vi "ArrayToExcelColumns.vi"(8 "error in (no error)":errorcluster, 9 "start row":i32, 10 "ArrayData":string[](array[string]), 11 "report in":refnum<class "NI_report.lvclass">) -> (0 "error in (no error) 2":errorcluster, 3 "report in 2":refnum<class "NI_report.lvclass">)   [LabVIEW 2012]
uses:
  <vilib>/Utility/NIReport.llb/NI_report.lvclass
  <vilib>/Utility/NIReport.llb/Excel/NI_Excel.lvclass
panel:
  in  "?":cluster{"start row":i32, "start column":i32}
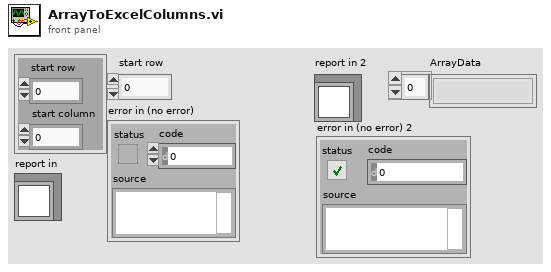
[diagram p1: front panel]
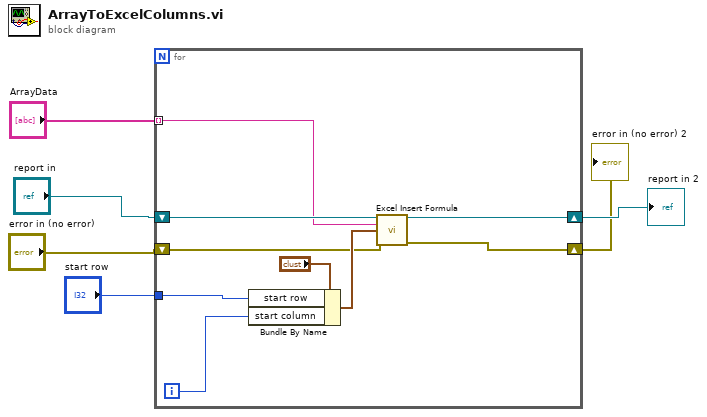
[diagram p0: block diagram]
diagram:
  n1 = for {
    tunnel: "start row" -> [w13]
    shift-right: [w11] -> w2
    shift-left: "report in" -> [w9]
    shift-right: [w10] -> w1
    shift-left: "error in (no error)" -> [w8]
    tunnel: "ArrayData" -> [w7] mode=indexing
    i -> [w14]
    n2 = Bundle By Name(cluster="?", "start row"=w13, "start column"=w14) -> (w12:cluster{"start row":i32, "start column":i32})
    n3 = call <vilib>:"Excel Insert Formula.vi"("report in"=w9, "formula"=w7, "start (0, 0)"=w12, "error in (no error)"=w8) -> ("report out"=w11:refnum<class "NI_report.lvclass">, "error out"=w10:errorcluster)  [unwired: 10 in]
  }
  "report in 2" <- w2
  "error in (no error) 2" <- w1
